vi "Facade.vi"(0 "Data In":T4, 2 "Display State In":T2, 3 "Container State":T3) -> (6 "Data Out":T4, 7 "Display State Out":T2, 8 "Action":T1)   [LabVIEW 2015, in "Editable I-O Listbox.xctl"]
uses:
  Editable I-O Listbox.xctl
  Data.ctl
  <vilib>/_xctls/Container State.ctl
  State.ctl
  <vilib>/_xctls/Action.ctl
  <vilib>/_xctls/XControlSupport.lvlib
panel:
  in  "Delete":bool
  in  "Insert":bool
  out "Delete (signal)":bool
  in  "Listbox":i32(listbox) caption="Outputs"
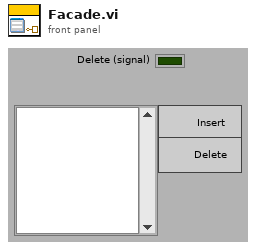
[diagram p1: front panel]
types:
  T1 = typedef "XControlSupport.lvlib/Action.ctl" = cluster{"Data Changed?":bool, "State Changed?":bool, "Action Name":string}
  T2 = typedef "Editable I-O Listbox.xctl/State.ctl" = cluster{"Rename?":bool, "Mandatory":string[]}
  T3 = typedef "XControlSupport.lvlib/Container State.ctl" = cluster{"Indicator?":bool, "Run Mode?":bool, " Refnum":refnum<vi>}
  T4 = typedef "Editable I-O Listbox.xctl/Data.ctl" = string[]
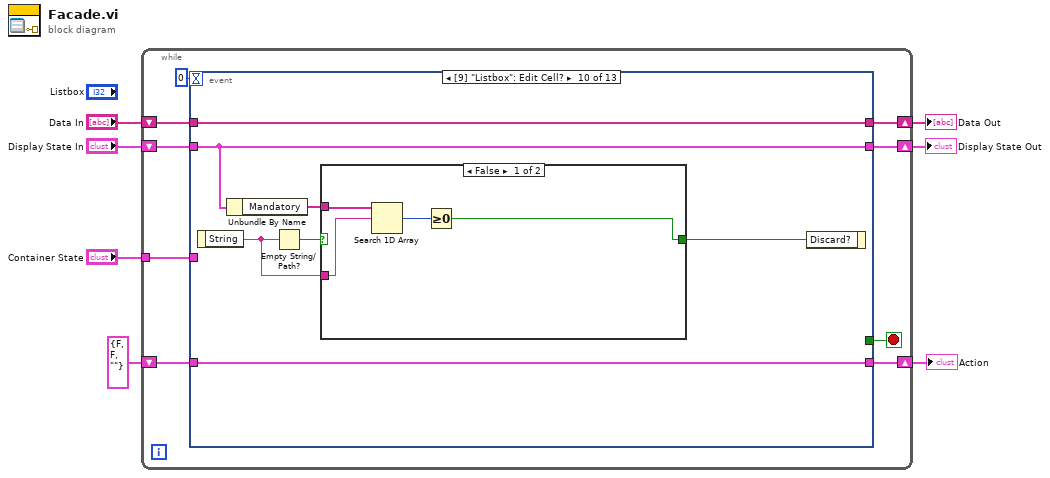
[diagram p0: block diagram]
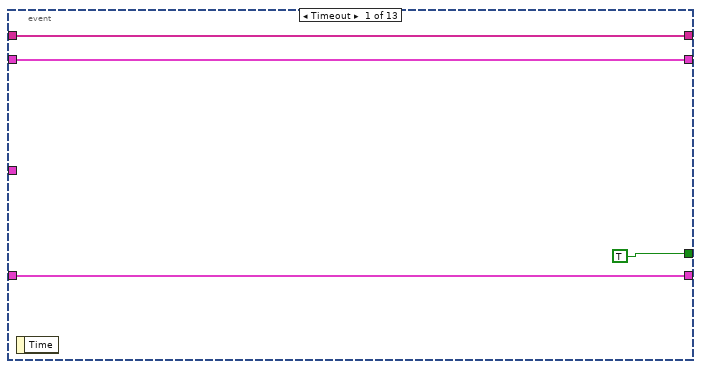
[diagram p2: hidden frame]
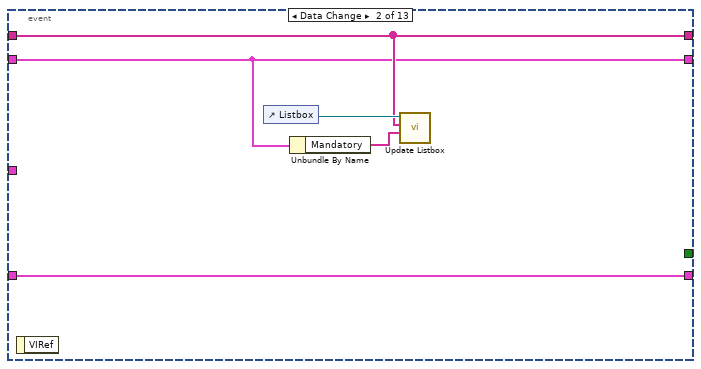
[diagram p3: hidden frame]
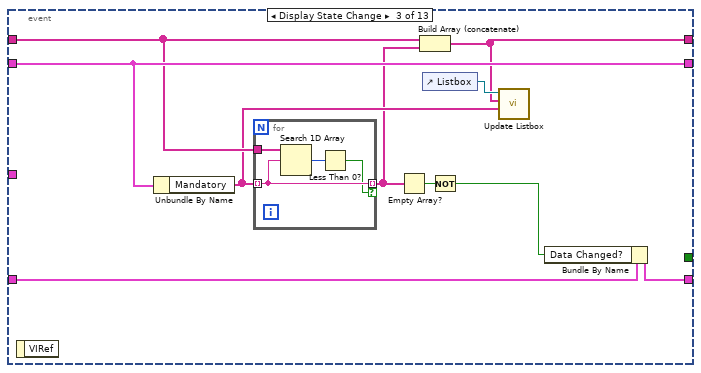
[diagram p4: hidden frame]
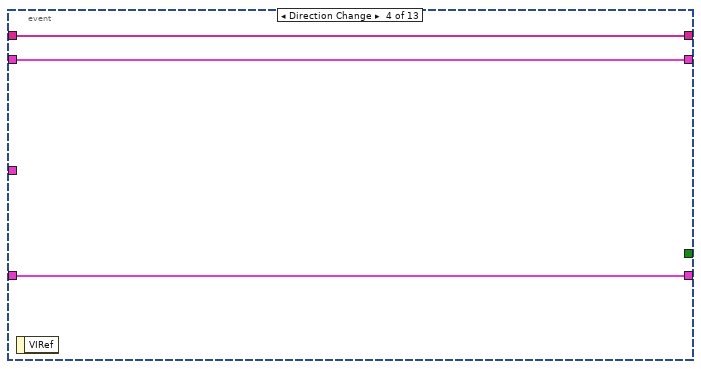
[diagram p5: hidden frame]
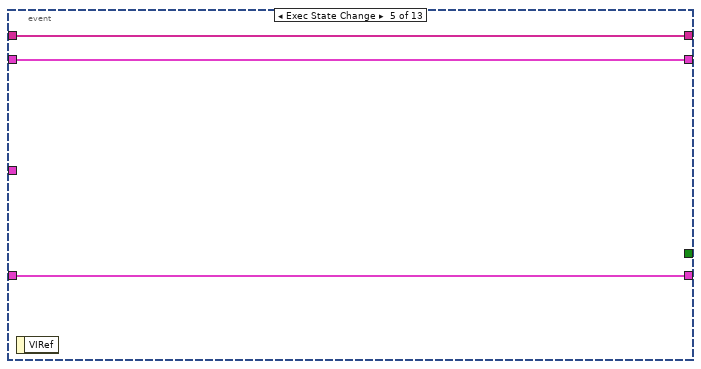
[diagram p6: hidden frame]
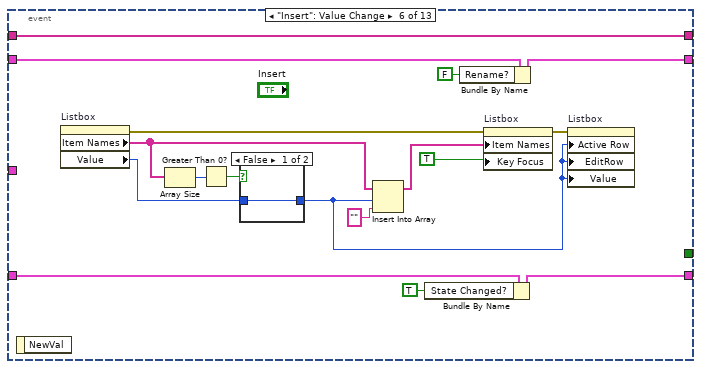
[diagram p7: hidden frame]
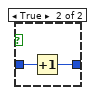
[diagram p8: hidden frame]
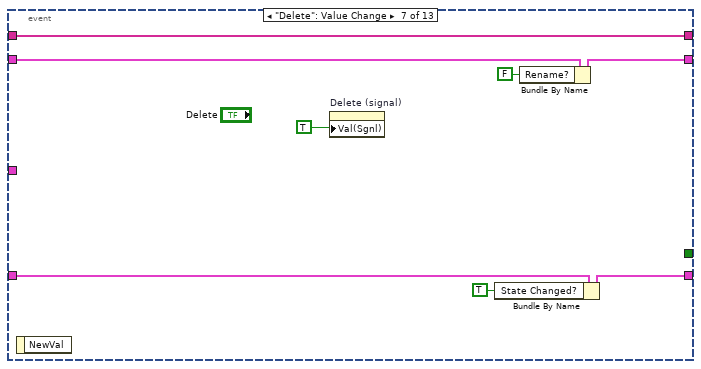
[diagram p9: hidden frame]
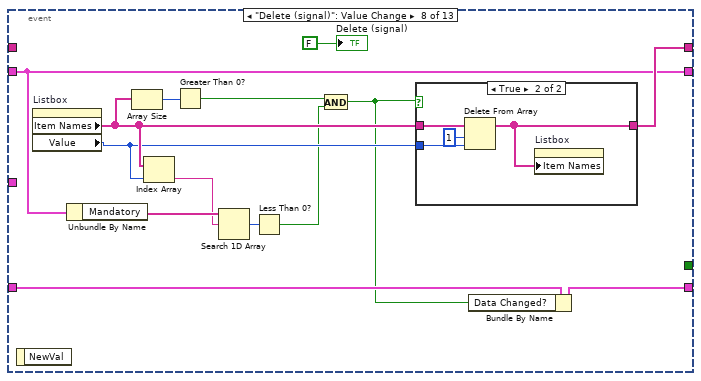
[diagram p10: hidden frame]
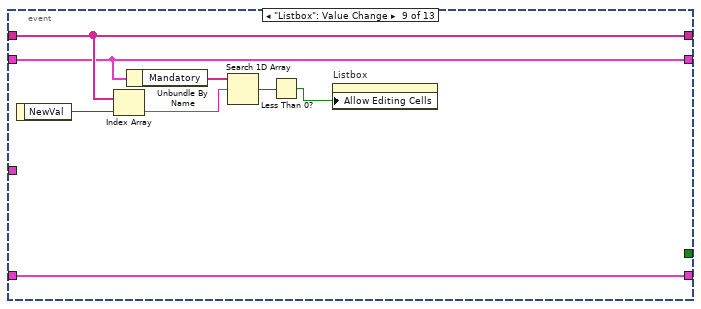
[diagram p12: hidden frame]
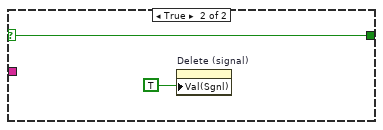
[diagram p13: hidden frame]
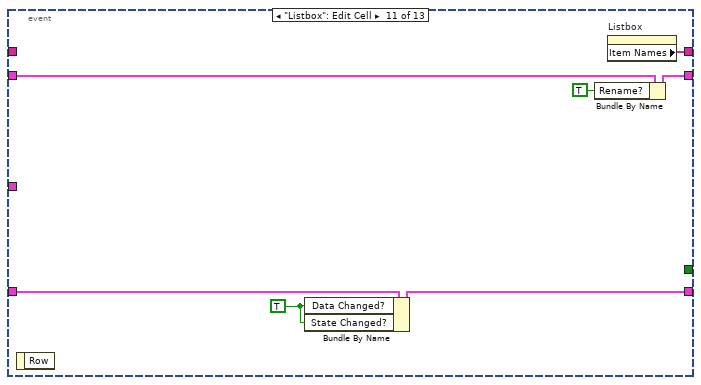
[diagram p14: hidden frame]
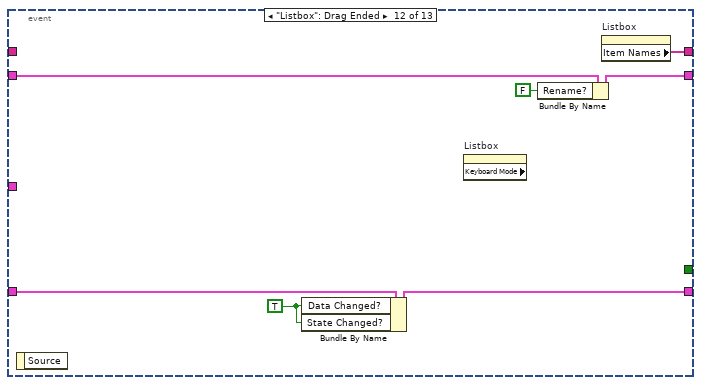
[diagram p15: hidden frame]
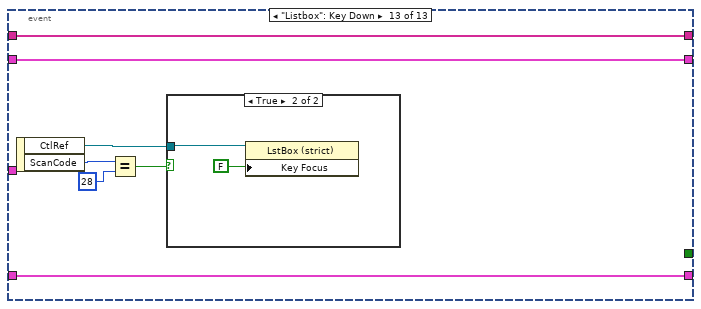
[diagram p16: hidden frame]
diagram:
  n1 = while {
    shift-right: [w15] -> w4
    shift-left: "Display State In" -> [w16]
    tunnel: "Container State" -> [w12]
    shift-right: [w10] -> w7
    shift-left: "Data In" -> [w11]
    shift-right: [w8] -> w2
    shift-left: T1 {"Data Changed?"=FALSE, "State Changed?"=FALSE, "Action Name"=""} ("Action") -> [w9]
    stop <- w14 stop-if-true
    n2 = event shown="[9] \"Listbox\": Edit Cell?" {
      selector: _ -> [_ _ _ _ _ _ _ _ _ _ _ _ _]
      dyn-events: _ -> [_ _ _ _ _ _ _ _ _ _ _ _ _]
      timeout: 0 -> [_ _ _ _ _ _ _ _ _ _ _ _ _]
      tunnel: w16 -> [w18 w22 w34 w42 w45 w53 w72 w81 w97 w102 w119 w126 w133]
      tunnel: [w18 w22 w34 w42 w45 w49 w69 w81 w97 w102 w115 w123 w133] -> w15
      tunnel: [TRUE _ _ _ _ _ _ _ _ _ _ _ _] -> w14
      tunnel: w12 -> [_ _ _ _ _ _ _ _ _ _ _ _ _]
      tunnel: w11 -> [w17 w23 w33 w41 w44 w55 w73 _ w99 w107 _ _ w134]
      tunnel: [w17 w23 w31 w41 w44 w55 w73 w84 w99 w107 w118 w127 w134] -> w10
      tunnel: [w19 w25 w29 w40 w43 w47 w67 w86 w100 w106 w117 w124 w132] -> w8
      tunnel: w9 -> [w19 w25 w35 w40 w43 w54 w71 w87 w100 w106 w120 w125 w132]
      event Timeout {
        n3 = event-data() -> ()  [unwired: 1 in, 1 out]
      }
      event Data Change {
        n4 = event-data() -> ()  [unwired: 1 in, 1 out]
        n5 = control-ref of="Listbox"() -> (w24:refnum<vi>)
        n6 = Unbundle By Name(w22) -> ("Mandatory"=w21:string[])
        n7 = call "Update Listbox.vi"("Mandatory"=w21, "Data In"=w23, "ListBox in"=w24) -> ()  [unwired: 7 in, 2 out]
      }
      event Display State Change {
        n8 = event-data() -> ()  [unwired: 1 in, 1 out]
        n9 = Unbundle By Name(w34) -> ("Mandatory"=w30:string[])
        n10 = for {
          tunnel: w30 -> [w37] mode=indexing
          tunnel: w33 -> [w39]
          tunnel: [w37] -> w28 mode=indexing if=w36
          n11 = Search 1D Array(1D array=w39, element=w37) -> (index of element=w38:i32)  [unwired: 1 in]
          n12 = Less Than 0?(x=w38) -> (x < 0?=w36:bool)
        }
        n13 = Empty Array?(array=w28) -> (empty?=w27:bool)
        n14 = Build Array (concatenate)(w33, w28) -> (w31:T4)
        n15 = control-ref of="Listbox"() -> (w32:refnum<vi>)
        n16 = Not(x=w27) -> (.not. x?=w26:bool)
        n17 = call "Update Listbox.vi"("Mandatory"=w30, "Data In"=w31, "ListBox in"=w32) -> ()  [unwired: 7 in, 2 out]
        n18 = Bundle By Name(cluster=w35, "Data Changed?"=w26) -> (w29:T1)
      }
      event Direction Change {
        n19 = event-data() -> ()  [unwired: 1 in, 1 out]
      }
      event Exec State Change {
        n20 = event-data() -> ()  [unwired: 1 in, 1 out]
      }
      event "Insert": Value Change {
        n21 = event-data() -> ()  [unwired: 1 in, 1 out]
        n22 = property on="Listbox" class="LstBox (strict)"() -> (error out=w61:errorcluster, "Item Names"=w52:string[], "Value"=w57:i32)  [unwired: 2 in, 1 out]
        n23 = Array Size(array=w52) -> (size(s)=w51:i32)
        n24 = Greater Than 0?(x=w51) -> (x > 0?=w50:bool)
        n25 = case shown="False" w50 {
          tunnel: w57 -> [w63 w65]
          tunnel: [w63 w64] -> w56
          frame False {
          }
          frame True {
            n26 = Increment(x=w65) -> (x+1=w64:i32)
          }
        }
        n27 = Insert Into Array(array=w52, index=w56, new element="" ("new element/subarray")) -> (w60:string[])
        n28 = Bundle By Name(cluster=w54, "State Changed?"=TRUE) -> (w47:T1)
        n29 = Bundle By Name(cluster=w53, "Rename?"=FALSE) -> (w49:T2)
        n30 = property on="Listbox" class="LstBox (strict)"(error in=w61, "Item Names"=w60, "Key Focus"=TRUE) -> (error out=w58:errorcluster)  [unwired: 1 in, 1 out]
        n31 = property on="Listbox" class="LstBox (strict)"(error in=w58, "Active Row"=w56, "EditRow"=w56, "Value"=w56) -> ()  [unwired: 1 in, 2 out]
      }
      event "Delete": Value Change {
        n32 = event-data() -> ()  [unwired: 1 in, 1 out]
        n33 = property on="Delete (signal)" class="Bool (strict)"("Val(Sgnl)"=TRUE ("Value (Signaling)")) -> ()  [unwired: 2 in, 2 out]
        n34 = Bundle By Name(cluster=w71, "State Changed?"=TRUE) -> (w67:T1)
        n35 = Bundle By Name(cluster=w72, "Rename?"=FALSE) -> (w69:T2)
      }
      event "Delete (signal)": Value Change {
        n36 = event-data() -> ()  [unwired: 1 in, 1 out]
        n37 = property on="Listbox" class="LstBox (strict)"() -> ("Item Names"=w80:string[], "Value"=w79:i32)  [unwired: 2 in, 2 out]
        n38 = Unbundle By Name(w81) -> ("Mandatory"=w78:string[])
        n39 = Array Size(array=w80) -> (size(s)=w85:i32)
        n40 = Index Array(array=w80, index=w79) -> (element=w77:string)
        n41 = Greater Than 0?(x=w85) -> (x > 0?=w83:bool)
        n42 = Search 1D Array(1D array=w78, element=w77) -> (index of element=w75:i32)  [unwired: 1 in]
        n43 = Less Than 0?(x=w75) -> (x < 0?=w74:bool)
        n44 = And(x=w83, y=w74) -> (x .and. y?=w76:bool)
        n45 = case shown="True" w76 {
          tunnel: w80 -> [w88 w92]
          tunnel: w79 -> [_ w91]
          tunnel: [w88 w89] -> w84
          frame False {
          }
          frame True {
            n46 = Delete From Array(array=w92, length=1, index=w91) -> (array with subset deleted=w89:string[])  [unwired: 1 out]
            n47 = property on="Listbox" class="LstBox (strict)"("Item Names"=w89) -> ()  [unwired: 2 in, 2 out]
          }
        }
        n48 = Bundle By Name(cluster=w87, "Data Changed?"=w76) -> (w86:T1)
        "Delete (signal)" <- FALSE ("Delete (signal)")
      }
      event "Listbox": Value Change {
        n49 = event-data() -> ("NewVal"=w98:i32)  [unwired: 1 in]
        n50 = Index Array(array=w99, index=w98) -> (element=w95:string)
        n51 = Unbundle By Name(w97) -> ("Mandatory"=w96:string[])
        n52 = Search 1D Array(1D array=w96, element=w95) -> (index of element=w94:i32)  [unwired: 1 in]
        n53 = Less Than 0?(x=w94) -> (x < 0?=w93:bool)
        n54 = property on="Listbox" class="LstBox (strict)"("Allow Editing Cells"=w93) -> ()  [unwired: 2 in, 2 out]
      }
      event "Listbox": Edit Cell? {
        n55 = event-data() -> ("String"=w103:string)  [unwired: 1 in]
        n56 = Unbundle By Name(w102) -> ("Mandatory"=w101:string[])
        n57 = Empty String/Path?(string/path=w103) -> (empty?=w105:bool)
        n58 = case shown="False" w105 {
          selector: w105 -> [_ w113]
          tunnel: [w108 w113] -> w104
          tunnel: w103 -> [w110 _]
          tunnel: w101 -> [w111 _]
          frame False {
            n59 = Search 1D Array(1D array=w111, element=w110) -> (index of element=w109:i32)  [unwired: 1 in]
            n60 = Greater Or Equal To 0?(x=w109) -> (x >= 0?=w108:bool)
          }
          frame True {
            n61 = property on="Delete (signal)" class="Bool (strict)"("Val(Sgnl)"=TRUE ("Value (Signaling)")) -> ()  [unwired: 2 in, 2 out]
          }
        }
        n62 = event-data("Discard?"=w104) -> ()  [unwired: 1 in, 1 out]
      }
      event "Listbox": Edit Cell {
        w116 = TRUE ("Data Changed?")
        n63 = event-data() -> ()  [unwired: 1 in, 1 out]
        n64 = Bundle By Name(cluster=w120, "Data Changed?"=w116, "State Changed?"=w116) -> (w117:T1)
        n65 = Bundle By Name(cluster=w119, "Rename?"=TRUE) -> (w115:T2)
        n66 = property on="Listbox" class="LstBox (strict)"() -> ("Item Names"=w118:string[])  [unwired: 2 in, 2 out]
      }
      event "Listbox": Drag Ended {
        w121 = TRUE ("Data Changed?")
        n67 = event-data() -> ()  [unwired: 1 in, 1 out]
        n68 = Bundle By Name(cluster=w125, "Data Changed?"=w121, "State Changed?"=w121) -> (w124:T1)
        n69 = property on="Listbox" class="LstBox (strict)" props=["Keyboard Mode"]() -> ()  [unwired: 2 in, 3 out]
        n70 = Bundle By Name(cluster=w126, "Rename?"=FALSE) -> (w123:T2)
        n71 = property on="Listbox" class="LstBox (strict)"() -> ("Item Names"=w127:string[])  [unwired: 2 in, 2 out]
      }
      event "Listbox": Key Down {
        n72 = event-data() -> ("CtlRef"=w129:refnum<vi>, "ScanCode"=w131:i16)  [unwired: 1 in]
        n73 = Equal?(x=w131, y=i16 28) -> (x = y?=w128:bool)
        n74 = case shown="True" w128 {
          tunnel: w129 -> [_ w136]
          frame False {
          }
          frame True {
            n75 = property class="LstBox (strict)"(reference=w136, "Key Focus"=FALSE) -> ()  [unwired: 1 in, 2 out]
          }
        }
      }
    }
  }
  "Display State Out" <- w4
  "Data Out" <- w7
  "Action" <- w2
